vi "NI 9208 Getting Started (Host).vi"(5 "RIO Device":T3="RIO0::INSTR") -> ()   [LabVIEW 2015]
doc: "This VI runs on the host device. The host can be a Windows PC or Real-Time target. The example downloads and runs an FPGA VI that continuously reads single point values from all 16 channels of a NI 9208 module."
uses:
  <vilib>/userdefined/High Color/nirio_resource_hc.ctl
  <vilib>/LabVIEW Targets/FPGA/cRIO/shared/nicrio_ModuleControls/nicrio_BasicConversionTime.ctl
  <vilib>/FPGAPlugInAG/cRIO-9031/niLvFpga_Open_cRIO-9031.vi
  <vilib>/rvi/interface/common/dynamic/niFpgaDynamicAddResources.vi
  <vilib>/Utility/error.llb/Error Cluster From Error Code.vi
  <vilib>/rvi/errors/niLvFpgaAdjustHostInterfaceError.vi
  <vilib>/FPGAPlugInAG/Dynamic/niLvFpga_Run_Dynamic.vi
  <vilib>/RVI Host/nirviSupport.llb/nirviErrorClusterFromErrorCode.vi
  <vilib>/FPGAPlugInAG/Dynamic/niLvFpga_Close_Dynamic.vi
  <vilib>/rvi/interface/nirviOpenFPGA/nirviOpenFPGA.xnode
  FPGA Bitfiles/W&RDArabia_FPGATarget_NI9208GettingSta_KylPh3mhQz8.lvbitx
  FPGA/NI 9208 Getting Started (FPGA).vi
  <vilib>/rvi/interface/nirviReadWriteControl/nirviReadWriteControl.xnode
  <vilib>/rvi/interface/nirviMethod/nirviMethod.xnode
  <vilib>/rvi/interface/nirviCloseFPGA/nirviCloseFPGA.xnode
  NiFpgaLv.dll
  <vilib>/rvi/interface/Simulation/niFpgaSimulationCallBeginRW.vi
  <vilib>/rvi/interface/nirviMethod/StockFPGA_InlinedMethodWaitForSingleIRQ.vi
  <vilib>/FPGAPlugInAG/Dynamic/niLvFpga_WaitOnIrq_Dynamic.vi
  <vilib>/FPGAPlugInAG/Dynamic/niLvFpga_AcknowledgeIrq_Dynamic.vi
panel:
  out "FPGA Error out":errorcluster
  out "Host Error out":errorcluster
  out "FPGA data transfer timed out":bool
  out "Analog Input":T1(graph)
  in  "Conversion Time":T2=enum."High Resolution"
  in  "Update":bool
  in  "stop":bool
  # "Overview: This example downloads and runs an FPGA VI that continuously reads single point values from 4 out of 16 channels of an NI 9208 module.\nRequirements: LabVIEW Full Development System, LV FPGA, and NI RIO\nInstructions: \n1) Modify the timing parameters if desired . It may also be changed during run-time using the \"Update\" button.\n2) Run the VI"
  # "Resource Parameters"
  # "Timing Parameters"
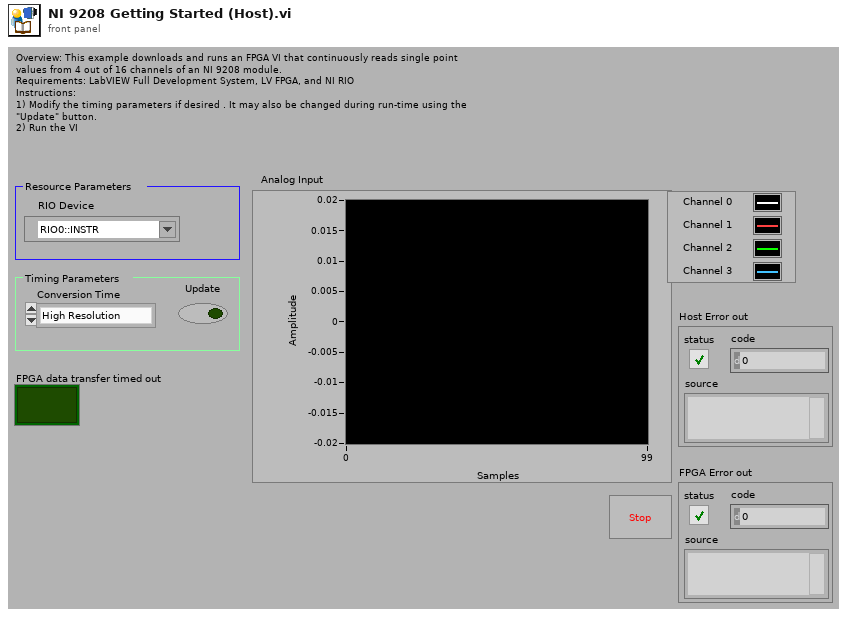
[diagram p1: front panel]
types:
  T1 = cluster{"Current Data[0]":dbl, "Current Data[1]":dbl, "Current Data[2]":dbl, "Current Data[3]":dbl, "Current Data[4]":dbl, "Current Data[5]":dbl, "Current Data[6]":dbl, "Current Data[7]":dbl, "Current Data[8]":dbl, "Current Data[9]":dbl, "Current Data[10]":dbl, "Current Data[11]":dbl, "Current Data[12]":dbl, "Current Data[13]":dbl, "Current Data[14]":dbl, "Current Data[15]":dbl}
  T2 = typedef "nicrio_BasicConversionTime.ctl" = enum8{"High Speed", "High Resolution"}
  T3 = typedef "nirio_resource_hc.ctl" = tag
  T4 = cluster{"Current Data[0]":fxp<+/-,24,-4>, "Current Data[1]":fxp<+/-,24,-4>, "Current Data[2]":fxp<+/-,24,-4>, "Current Data[3]":fxp<+/-,24,-4>, "Current Data[4]":fxp<+/-,24,-4>, "Current Data[5]":fxp<+/-,24,-4>, "Current Data[6]":fxp<+/-,24,-4>, "Current Data[7]":fxp<+/-,24,-4>, "Current Data[8]":fxp<+/-,24,-4>, "Current Data[9]":fxp<+/-,24,-4>, "Current Data[10]":fxp<+/-,24,-4>, "Current Data[11]":fxp<+/-,24,-4>, "Current Data[12]":fxp<+/-,24,-4>, "Current Data[13]":fxp<+/-,24,-4>, "Current Data[14]":fxp<+/-,24,-4>, "Current Data[15]":fxp<+/-,24,-4>}
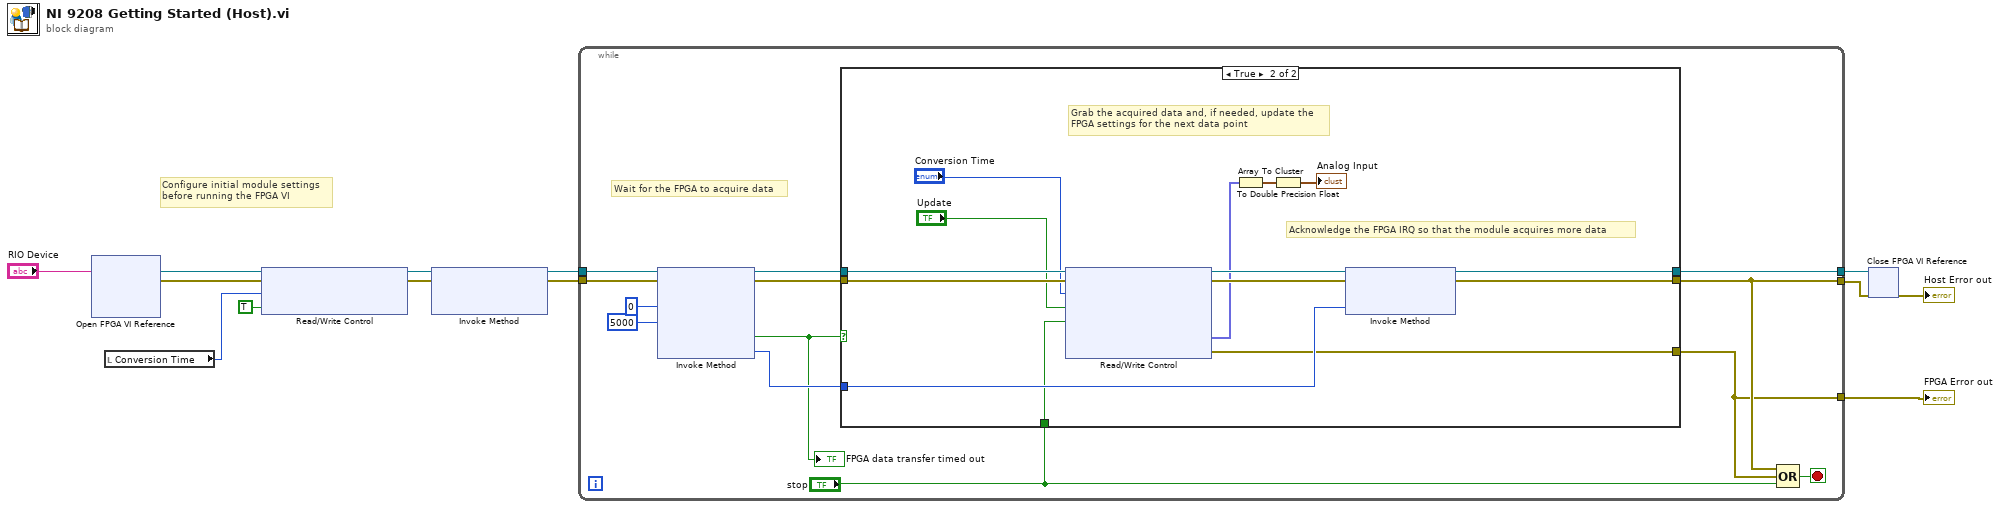
[diagram p0: block diagram]
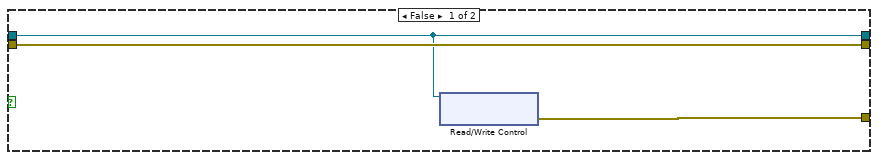
[diagram p2: hidden frame]
diagram:
  # "Configure initial module settings\nbefore running the FPGA VI"
  n1 = xnode "Open FPGA VI Reference"("resource name"="RIO Device") -> ("FPGA VI Reference Out"=w6:refnum<k20>, "error out"=w5:errorcluster)  [unwired: 1 in]
  n2 = local read "Conversion Time"() -> (w4:T2)
  n3 = xnode "Read/Write Control"("FPGA VI Reference In"=w6, "error in"=w5, "Conversion Time"=w4, "Update Conversion Time"=TRUE) -> ("FPGA VI Reference Out"=w7:refnum<k20>, "error out"=w8:errorcluster)
  n4 = xnode "Invoke Method"("FPGA VI Reference In"=w7, "error in"=w8) -> ("FPGA VI Reference Out"=w10:refnum<k20>, "error out"=w9:errorcluster)  [unwired: 1 in]
  n5 = while {
    tunnel: w10 -> [w26]
    tunnel: w9 -> [w25]
    tunnel: [w20] -> w12
    tunnel: [w17] -> w11
    tunnel: [w16] -> w3
    stop <- w18 stop-if-true
    # "Wait for the FPGA to acquire data"
    n6 = xnode "Invoke Method"("FPGA VI Reference In"=w26, "error in"=w25, "IRQ Number(s)"=0, "Timeout (ms)"=5000 ("timeout (ms)(-1 for no timeout)")) -> ("FPGA VI Reference Out"=w22:refnum<k20>, "error out"=w21:errorcluster, "Timed Out"=w14:bool, "IRQ(s) Asserted"=w19:i32)
    "FPGA data transfer timed out" <- w14
    n7 = case shown="True" w14 {
      tunnel: w22 -> [w27 w43]
      tunnel: w21 -> [w28 w42]
      tunnel: [w27 w40] -> w20
      tunnel: w19 -> [_ w39]
      tunnel: "stop" -> [_ w35]
      tunnel: [w29 w37] -> w16
      tunnel: [w28 w36] -> w17
      frame False {
        n8 = xnode "Read/Write Control"("FPGA VI Reference In"=w27) -> ("FPGA Error Out"=w29:errorcluster)  [unwired: 1 in, 2 out]
      }
      frame True {
        # "Acknowledge the FPGA IRQ so that the module acquires more data"
        # "Grab the acquired data and, if needed, update the \nFPGA settings for the next data point"
        n9 = xnode "Read/Write Control"("FPGA VI Reference In"=w43, "error in"=w42, "Conversion Time"="Conversion Time", "Update Conversion Time"="Update", "Stop"=w35) -> ("FPGA VI Reference Out"=w41:refnum<k20>, "error out"=w38:errorcluster, "Current Data"=w32:fxp<+/-,24,-4>[], "FPGA Error Out"=w37:errorcluster)
        n10 = Array To Cluster(array=w32) -> (cluster=w33:T4)
        n11 = To Double Precision Float(number=w33) -> (double precision float=→"Analog Input":T1)
        n12 = xnode "Invoke Method"("FPGA VI Reference In"=w41, "error in"=w38, "IRQ Number(s)"=w39) -> ("FPGA VI Reference Out"=w40:refnum<k20>, "error out"=w36:errorcluster)
      }
    }
    n13 = Compound Arithmetic op=OR(w17, w16, "stop") -> (w18:bool)
  }
  "FPGA Error out" <- w3
  n14 = xnode "Close FPGA VI Reference"("FPGA VI Reference In"=w12, "error in"=w11) -> ("error out"=→"Host Error out":errorcluster)
